vi "Write timeToBlindSpot_min.vi"(8 "error in (no error)":errorcluster, 10 "timeToBlindSpot_min":dbl[unit], 11 "Zenith in":refnum<class "Zenith.lvclass">) -> (0 "error out":errorcluster, 3 "Zenith out":refnum<class "Zenith.lvclass">)   [LabVIEW 2014, in "TCSDataDefinitions.lvlib" / "TCSPublicStatus.lvlib" / "Limits.lvlib" / "Zenith.lvclass"]
uses:
  Zenith.lvclass
  Zenith.lvclass/Zenith.ctl
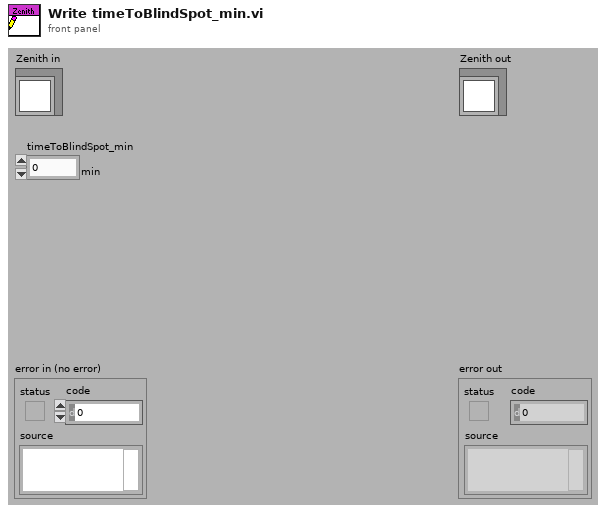
[diagram p1: front panel]
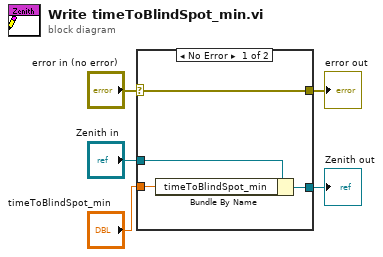
[diagram p0: block diagram]
diagram:
  n1 = case shown="No Error" "error in (no error)" {
    selector: "error in (no error)" -> [w9 w10]
    tunnel: [w9 w10] -> w4
    tunnel: [w7 w11] -> w2
    tunnel: "Zenith in" -> [w8 w11]
    tunnel: "timeToBlindSpot_min" -> [w6 _]
    frame No Error {
      n2 = Bundle By Name(cluster=w8, "timeToBlindSpot_min"=w6) -> (w7:refnum<class "Zenith.lvclass">)
    }
    frame Error {
    }
  }
  "error out" <- w4
  "Zenith out" <- w2
